vi "Open Instrument.vi"(8 "error in (no error)":errorcluster, 11 "VNA":refnum<class "VNA.lvclass">) -> (0 "error out":errorcluster, 3 "VNA out":refnum<class "VNA.lvclass">)   [LabVIEW 2016, in "VNA.lvclass"]
uses:
  VNA.lvclass
  VNA.lvclass/VNA.ctl
  P:/users1/Dengyu/Agilent 87XX Series/Agilent 87XX Series.lvlib
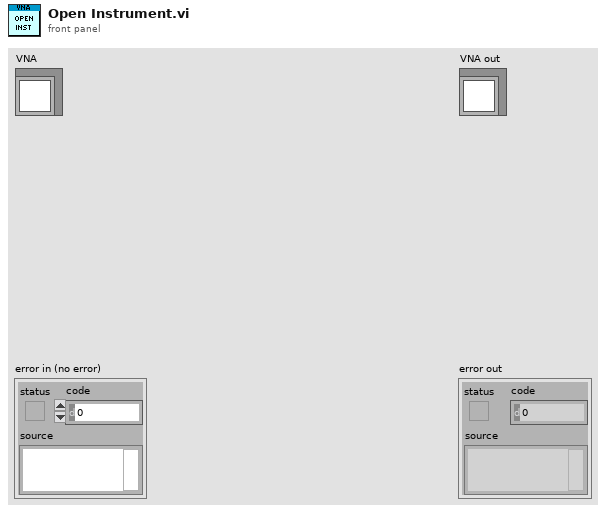
[diagram p1: front panel]
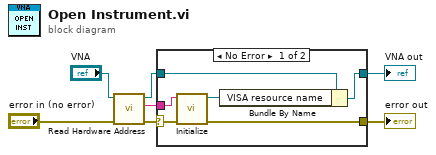
[diagram p0: block diagram]
diagram:
  n1 = call-dynamic "Read Hardware Address.vi"("error in (no error)"="error in (no error)", "Instrument in"="VNA") -> ("error out"=w3:errorcluster, "Hardware Address"=w5:string, "Instrument out"=w2:refnum<class "VNA.lvclass">)  [unwired: 7 in]
  n2 = case shown="No Error" w3 {
    selector: w3 -> [w11 w15]
    tunnel: [w13 w15] -> w7
    tunnel: w5 -> [w12 _]
    tunnel: w2 -> [w10 w14]
    tunnel: [w8 w14] -> w1
    frame No Error {
      n3 = call "Initialize.vi"("error in (no error)"=w11, "VISA resource name"=w12) -> ("error out"=w13:errorcluster, "VISA resource name out"=w9:refnum<visa-resource-name>)  [unwired: 8 in]
      n4 = Bundle By Name(cluster=w10, "VISA resource name"=w9) -> (w8:refnum<class "VNA.lvclass">)
    }
    frame Error {
    }
  }
  "error out" <- w7
  "VNA out" <- w1
